vi "Money Entered.vi"(8 "error in (no error)":errorcluster, 10 "New Balance":u32) -> (0 "error out":errorcluster)   [LabVIEW 2019, in "Money.lvlib"]
doc: "The operator has entered some money (in pence)\n_____\nCreated using Delacor QMH Event Scripter 4.2.1.88."
uses:
  Money.lvlib
  Money Entered Argument--cluster.ctl
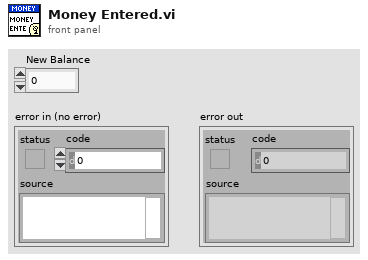
[diagram p1: front panel]
types:
  T1 = typedef "Money.lvlib/Money Entered Argument--cluster.ctl" = cluster{"New Balance":u32}
  T2 = typedef "Money.lvlib/Broadcast Events--cluster.ctl" = cluster{"Module Did Init":refnum<user-event>, "Status Updated":refnum<user-event>, "Error Reported":refnum<user-event>, "Module Did Stop":refnum<user-event>, "Update Module Execution Status":refnum<user-event>, "Money Entered":refnum<user-event>, "Money Refunded":refnum<user-event>}
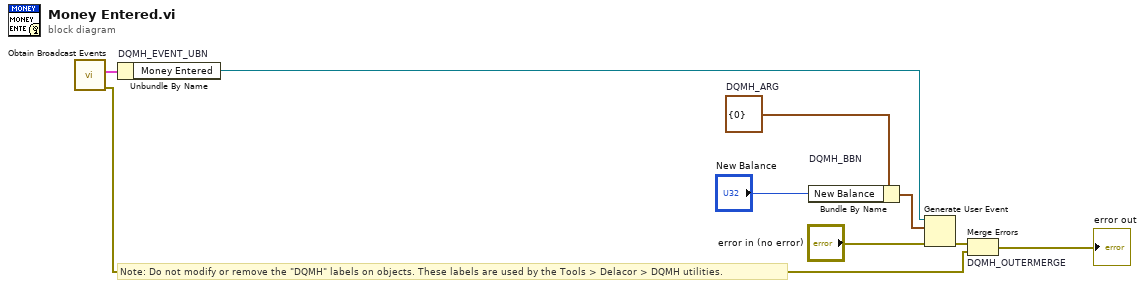
[diagram p0: block diagram]
diagram:
  w4 = T1 {"New Balance"=0}  # DQMH_ARG
  # "Note: Do not modify or remove the \"DQMH\" labels on objects. These labels are used by the Tools > Delacor > DQMH utilities."
  n1 = call "Obtain Broadcast Events.vi"() -> ("error out"=w2:errorcluster, "Money Broadcast Events"=w1:T2)  [unwired: 10 in]
  n2 = Unbundle By Name "DQMH_EVENT_UBN"(w1) -> ("Money Entered"=w6:refnum<user-event>)
  n3 = Bundle By Name "DQMH_BBN"(cluster=w4, "New Balance"="New Balance") -> (w7:T1)
  n4 = Generate User Event(user event=w6, event data cluster=w7, error in="error in (no error)") -> (error out=w5:errorcluster)  [unwired: 1 in, 1 out]
  n5 = Merge Errors "DQMH_OUTERMERGE"(w5, w2) -> (→"error out":errorcluster)
